vi "Test Float Param.vi"() -> ()   [LabVIEW 2020]
uses:
  VoiceMeeterRemote/VoiceMeeterRemote/VoiceMeeterRemote.lvclass
panel:
  out "Parameters Dirty?":bool
  out "Value":sgl
  out "error out":errorcluster
  in  "Parameter Name":string="Strip[0].Gain"
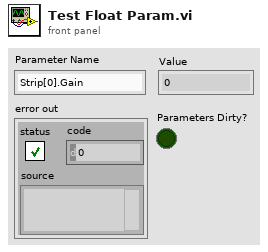
[diagram p1: front panel]
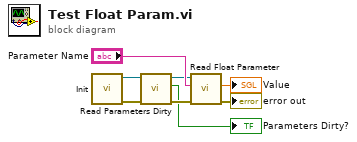
[diagram p0: block diagram]
diagram:
  n1 = call "Init.vi"() -> ("error out"=w4:errorcluster, "VoiceMeeterRemote out"=w5:refnum<class "VoiceMeeterRemote.lvclass">)  [unwired: 9 in, 1 out]
  n2 = call "Read Parameters Dirty.vi"("error in (no error)"=w4, "VoiceMeeterRemote in"=w5) -> ("error out"=w3:errorcluster, "Parameters Dirty?"=→"Parameters Dirty?":bool, "VoiceMeeterRemote out"=w2:refnum<class "VoiceMeeterRemote.lvclass">)  [unwired: 7 in]
  n3 = call "Read Float Parameter.vi"("error in (no error)"=w3, "Parameter Name"="Parameter Name", "VoiceMeeterRemote in"=w2) -> ("error out"=→"error out":errorcluster, "Value"=→"Value":sgl)  [unwired: 6 in, 1 out]
